vi "LEBITplc.CheckMonLL.vi"(1 "i attribute in":T1, 3 "index":i32, 7 "MonValuePLC":string) -> (15 "Monvalue":dbl)   [LabVIEW 2014, in "LEBITplc.lvlib"]
uses:
  LEBITplc.lvlib
  CS_Core/CSSystem/CoreDefs/CoreDefs.call_type.ctl
  CS_Core/BaseProcess/BaseProcess.descriptor string definition.ctl
  CS_Core/CSSystem/CoreDefs/CoreDefs.rawDataType.ctl
  LEBITplc.i attribute.ctl
  CSlibraries/UtilityLib/UtilityLib.valueStatus.ctl
  CS_Core/CSSystem/CoreLib/CoreLib.string 2 byte array.vi
  CS_Core/CSSystem/CoreLib/CoreLib.byte array 2 double.vi
  CS_Core/CSSystem/CoreLib/CoreLib.lvlib
  CSlibraries-extern/DimLVEvent/LVDimInterface/LVDimInterface.lvlib
  CSlibraries/UtilityLib/UtilityLib.lvlib
  CS_Core/BaseProcess/BaseProcess.lvlib
panel:
  in  "call cluster in":T2={"Object"="", "Selector"="", "CallType"=enum."synchronous", "Async Object"="", "Async Selector"="", "Data Descriptor"="", "Data"=[], "Error #"=0, "Expire"=0}
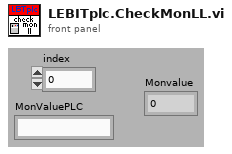
[diagram p1: front panel]
types:
  T1 = typedef "LEBITplc.lvlib/LEBITplc.i attribute.ctl" = cluster{"LLFLocation":string, "SetFileLocation":string, "nickNames":string[], "setValuePLCServiceID":i32[], "GUIServiceID":i32[], "monValuePLC":string[], "SetValueServiceID":i32[], "MonValueServiceID":i32[], "SetValue":dbl[][], "SetValueMin":dbl[], "SetValueMax":dbl[], "SetValueInfoServiceID":i32[], "GUINames":string[], "ListOfBases":string[], "Scale":dbl[], "Offset":dbl[], "setValuePLC":string[], "BaseName":string[], "ScaleServiceID":i32[], "OffsetServiceID":i32[], "AllPLCValues":string[], "CondSpecialArray":string[][], "CondSpecialIndex":i32[], "CondSpecialMonValue":dbl[], "RecentlyChanged":i32[], "SetFileLocationID":i32, "Dependent-Monitors":string[][], "LastLoadedFiles":string[], "IonGuideCalibLocation":string, "Monitor Dependent":string[], "Special":string[], "PLC?":bool[], "Start Date":string, "ListOfBasesServiceID":i32, "SETRA VISA resource":refnum<visa-resource-name>}
  T2 = typedef "CoreDefs.call_type.ctl" = cluster{"Object":string, "Selector":string, "CallType":enum16{"simple", "synchronous", "asynchronous"}, "Async Object":string, "Async Selector":string, "Data Descriptor":T3, "Data":T4, "Error #":i32, "Expire":u32}
  T3 = typedef "BaseProcess.lvlib/BaseProcess.descriptor string definition.ctl" = string
  T4 = typedef "CoreDefs.rawDataType.ctl" = i8[]
  T5 = typedef "UtilityLib.lvlib/UtilityLib.valueStatus.ctl" = enum16{"no info available", "stand by/off", "on", "warning", "alarm/malfunction", "not implemented", "user action required", "important information", "system default", "control default", "indicator default", "button default"}
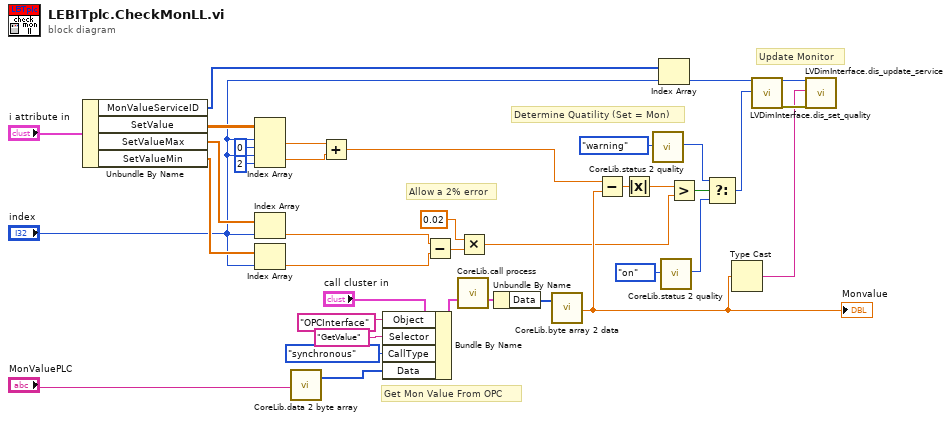
[diagram p0: block diagram]
diagram:
  # "Update Monitor"
  # "Allow a 2% error"
  # "Determine Quatility (Set = Mon)"
  # "Get Mon Value From OPC"
  n1 = Unbundle By Name("i attribute in") -> ("MonValueServiceID"=w12:i32[], "SetValue"=w11:dbl[][], "SetValueMax"=w6:dbl[], "SetValueMin"=w5:dbl[])
  n2 = Index Array(array=w11, index (row) #1="index", index (col) #1=0 ("disabled index (col)"), index (row) #2="index", index (col) #2=2 ("disabled index (col)")) -> (element #1=w10:dbl, element #2=w9:dbl)
  n3 = Index Array(array=w6, index="index") -> (element=w3:dbl)
  n4 = Index Array(array=w5, index="index") -> (element=w2:dbl)
  n5 = call-poly "CoreLib.data 2 byte array.vi"("string"="MonValuePLC") -> ("byteArray out"=w16:T4)  [unwired: 18 in]
  n6 = Add(x=w10, y=w9) -> (x+y=w37:dbl)
  n7 = Bundle By Name(cluster="call cluster in", "Object"="OPCInterface", "Selector"="GetValue" ("string"), "CallType"=enum16{"simple", "synchronous", "asynchronous"}."synchronous", "Data"=w16) -> (w13:T2)
  n8 = Subtract(x=w3, y=w2) -> (x-y=w24:dbl)
  n9 = call "CoreLib.call process.vi"("call cluster in"=w13) -> ("call cluster out"=w19:T2)  [unwired: 13 in, 1 out]
  n10 = Multiply(x=0.02 ("y"), y=w24) -> (x*y=w28:dbl)
  n11 = Unbundle By Name(w19) -> ("Data"=w20:T4)
  n12 = call-poly "CoreLib.byte array 2 data.vi"("byteArray"=w20) -> ("d64"=w35:dbl)  [unwired: 16 in, 2 out]
  "Monvalue" <- w35
  n13 = Subtract(x=w37, y=w35) -> (x-y=w25:dbl)
  n14 = Absolute Value(x=w25) -> (abs(x)=w27:dbl)
  n15 = call "CoreLib.status 2 quality.vi"("valueStatus"=UtilityLib.valueStatus."warning") -> ("quality"=w31:i32)  [unwired: 18 in]
  n16 = Index Array(array=w12, index="index") -> (element=w22:i32)
  n17 = call "CoreLib.status 2 quality.vi"("valueStatus"=UtilityLib.valueStatus."on") -> ("quality"=w30:i32)  [unwired: 18 in]
  n18 = Greater?(x=w27, y=w28) -> (0:w26:bool)
  n19 = Select(t=w31, s=w26, f=w30) -> (s? t:f=w32:i32)
  n20 = Type Cast(x=w35) -> (*(type *) &x=w34:string)  [unwired: 1 in]
  n21 = call "LVDimInterface.dis_set_quality.vi"("my_serviceID"=w22, "quality"=w32) -> ("my_serviceID (out)"=w33:i32, "error out"=w36:errorcluster)  [unwired: 16 in]
  n22 = call "LVDimInterface.dis_update_service.vi"("my_serviceID"=w33, "data"=w34, "error in (no error)"=w36) -> ()  [unwired: 14 in, 3 out]
